vi "Read distance type.vi"(8 "error in (no error)":errorcluster, 11 "KD Tree in":refnum<class "KD Tree.lvclass">) -> (0 "error out":errorcluster, 2 "distance type":T1 items=["EUCLIDEAN"=1, "MANHATTAN"=2, "MINKOWSKY"=3, "HIST INTERSECT"=5, "HELLINGER"=6, "CHI SQUARE"=7, "KULLBACK LEIBLER"=8], 3 "KD Tree out":refnum<class "KD Tree.lvclass">)   [LabVIEW 2020, in "KD Tree.lvlib" / "KD Tree.lvclass"]
uses:
  KD Tree.lvclass
  KD Tree.lvclass/KD Tree.ctl
  flann/Distance Type.ctl
  KD Tree.lvlib
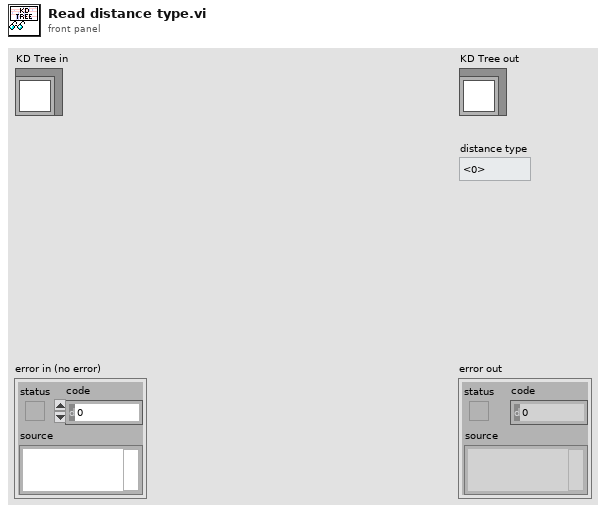
[diagram p1: front panel]
types:
  T1 = typedef "KD Tree.lvlib/Distance Type.ctl" = u32
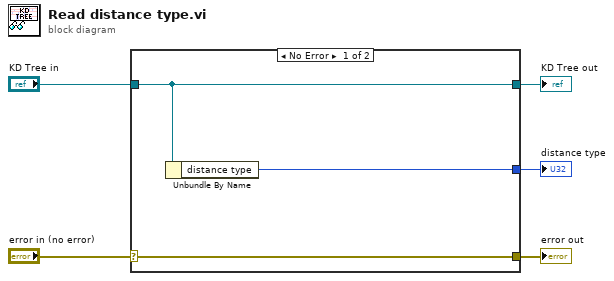
[diagram p0: block diagram]
diagram:
  n1 = case shown="No Error" "error in (no error)" {
    selector: "error in (no error)" -> [w8 w9]
    tunnel: [w8 w9] -> w4
    tunnel: [w7 w10] -> w2
    tunnel: "KD Tree in" -> [w7 w10]
    tunnel: [w6 _] -> w1
    frame No Error {
      n2 = Unbundle By Name(w7) -> ("distance type"=w6:T1)
    }
    frame Error {
    }
  }
  "error out" <- w4
  "KD Tree out" <- w2
  "distance type" <- w1
